vi "Reposition After.vi"(11 "Front Panel Objects":refnum<vi>[](array[refnum])) -> ()   [LabVIEW 2019, in "LSS.lvlib"]
doc: "Repositions front panel objects of example using LSS.\n\n<b>Inputs:</b>\n<b>Front Panel Objects</b> - Array of front panel controls that will have style applied to them."
uses:
  LSS.lvlib
  <vilib>/Utility/miscctls.llb/LVBoundsTypeDef.ctl
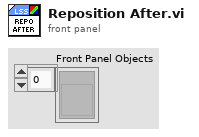
[diagram p1: front panel]
types:
  T1 = typedef "LVBoundsTypeDef.ctl" = cluster{"Width":u32, "Height":u32}
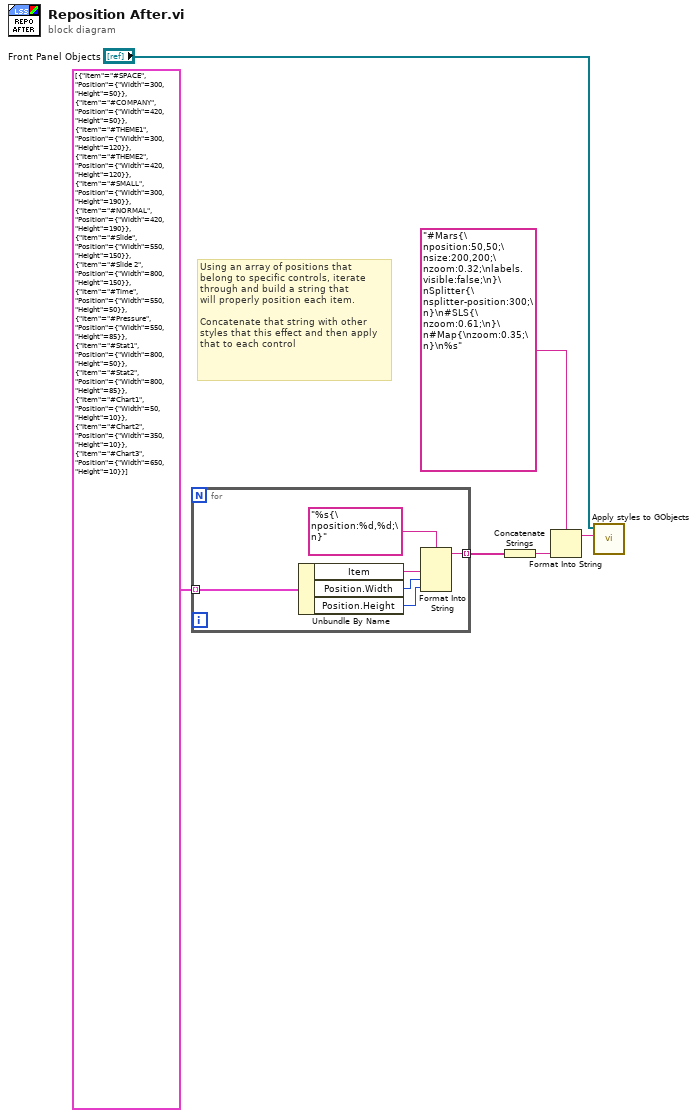
[diagram p0: block diagram]
diagram:
  # "Using an array of positions that\nbelong to specific controls, iterate\nthrough and build a string that\nwill properly position each item.\n\nConcatenate that string with other\nstyles that this effect and then apply\nthat to each control"
  n1 = for {
    tunnel: cluster{"Item":string, "Position":T1}[] [{"Item"="#SPACE", "Position"={"Width"=300, "Height"=50}}, {"Item"="#COMPANY", "Position"={"Width"=420, "Height"=50}}, {"Item"="#THEME1", "Position"={"Width"=300, "Height"=120}}, {"Item"="#THEME2", "Position"={"Width"=420, "Height"=120}}, {"Item"="#SMALL", "Position"={"Width"=300, "Height"=190}}, {"Item"="#NORMAL", "Position"={"Width"=420, "Height"=190}}, {"Item"="#Slide", "Position"={"Width"=550, "Height"=150}}, {"Item"="#Slide 2", "Position"={"Width"=800, "Height"=150}}, {"Item"="#Time", "Position"={"Width"=550, "Height"=50}}, {"Item"="#Pressure", "Position"={"Width"=550, "Height"=85}}, {"Item"="#Stat1", "Position"={"Width"=800, "Height"=50}}, {"Item"="#Stat2", "Position"={"Width"=800, "Height"=85}}, {"Item"="#Chart1", "Position"={"Width"=50, "Height"=10}}, {"Item"="#Chart2", "Position"={"Width"=350, "Height"=10}}, {"Item"="#Chart3", "Position"={"Width"=650, "Height"=10}}] -> [w12] mode=indexing
    tunnel: [w7] -> w3 mode=indexing
    n2 = Unbundle By Name(w12) -> ("Item"=w10:string, "Position.Width"=w9:u32, "Position.Height"=w8:u32)
    n3 = Format Into String(format string="%s{\nposition:%d,%d;\n}", w10, w9, w8) -> (resulting string=w7:string)  [unwired: 2 in, 1 out]
  }
  n4 = Concatenate Strings(w3) -> (w2:string)
  n5 = Format Into String(format string="#Mars{\nposition:50,50;\nsize:200,200;\nzoom:0.32;\nlabels.visible:false;\n}\nSplitter{\nsplitter-position:300;\n}\n#SLS{\nzoom:0.61;\n}\n#Map{\nzoom:0.35;\n}\n%s" ("String"), w2) -> (resulting string=w1:string)  [unwired: 2 in, 1 out]
  n6 = call "Apply styles to GObjects.vi"("Style Sheet"=w1, "Front Panel Objects"="Front Panel Objects") -> ()  [unwired: 8 in, 2 out]
